vi "stacksecuence.vi"() -> ()   [LabVIEW 2016]
panel:
  out "x-y":dbl
  out "Triangle":dynamicdata(graph)
  out "Sine":dynamicdata(graph)
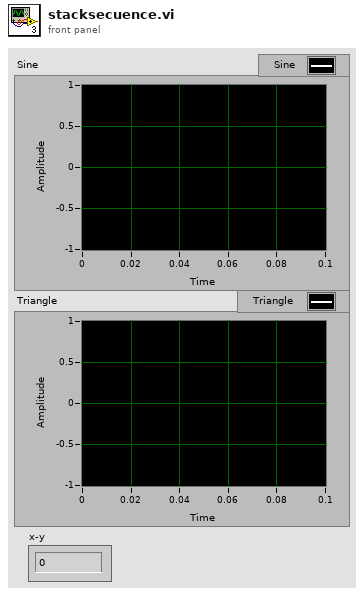
[diagram p1: front panel]
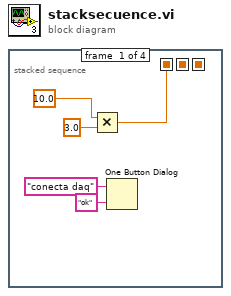
[diagram p0: block diagram]
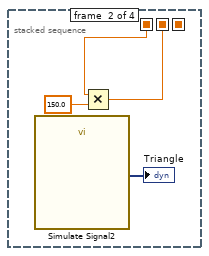
[diagram p2: hidden frame]
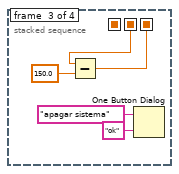
[diagram p3: hidden frame]
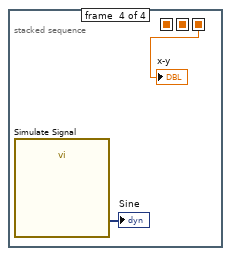
[diagram p4: hidden frame]
diagram:
  n1 = stacked-sequence {
    seq-local: [w2 _ _ _] -> [_ w7 _ _]
    seq-local: [_ w6 _ _] -> [_ _ w12 _]
    seq-local: [_ _ w10 _] -> [_ _ _ w15]
    frame #0 {
      n2 = Multiply(x=10.0, y=3.0) -> (x*y=w2:dbl)
      n3 = One Button Dialog(message="conecta daq", button name ("OK")="ok") -> ()  [unwired: 1 out]
    }
    frame #1 {
      n4 = call "Simulate Signal2"() -> ("Triangle"=→"Triangle":dynamicdata)  [unwired: 14 in, 1 out]
      n5 = Multiply(x=w7, y=150.0) -> (x*y=w6:dbl)
    }
    frame #2 {
      n6 = Subtract(x=w12, y=150.0) -> (x-y=w10:dbl)
      n7 = One Button Dialog(message="apagar sistema", button name ("OK")="ok") -> ()  [unwired: 1 out]
    }
    frame #3 {
      n8 = call "Simulate Signal"() -> ("Sine"=→"Sine":dynamicdata)  [unwired: 14 in, 1 out]
      "x-y" <- w15
    }
  }
